vi "Test_WriteValue_NoCaption_Error.vi"(8 "error in (no error)":errorcluster, 11 "TestCase in":refnum<class "TestTerminalCaptionBinding.lvclass">) -> (0 "error out":errorcluster, 3 "TestCase out":refnum<class "TestTerminalCaptionBinding.lvclass">)   [LabVIEW 2017, in "TestTerminalCaptionBinding.lvclass"]
uses:
  TestTerminalCaptionBinding.lvclass
  Source/Concrete/TerminalCaptionBinding/TerminalCaptionBinding.lvclass
  C:/Git/composed-transport/Source/ITransport/ITransport.lvclass
  Source/ITransport/ITransport.lvclass
panel:
  out "Return Error":errorcluster
  in  "Numeric":dbl
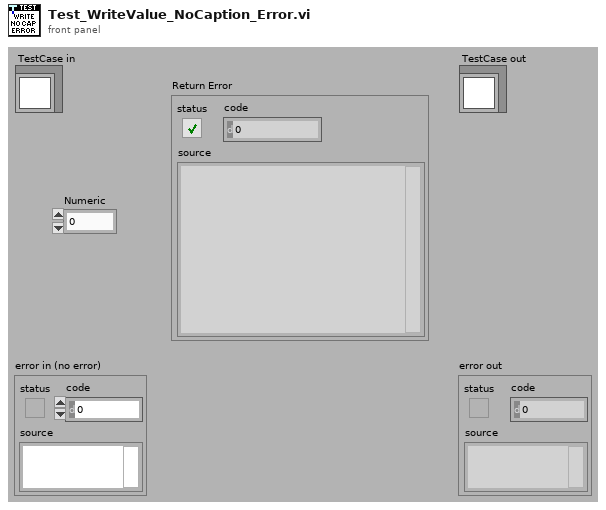
[diagram p1: front panel]
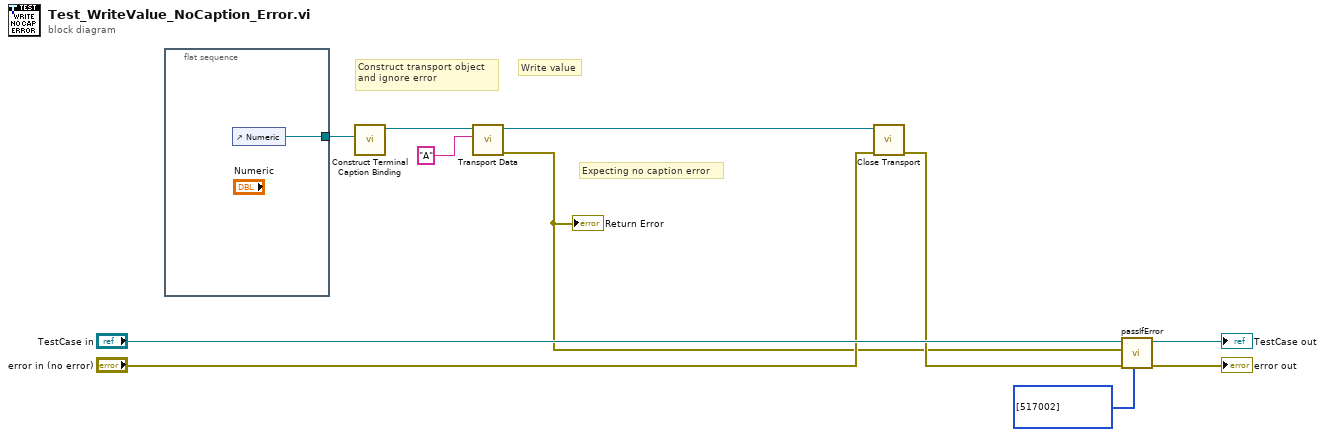
[diagram p0: block diagram]
diagram:
  # "Write value"
  # "Expecting no caption error"
  # "Construct transport object\nand ignore error"
  n1 = flat-sequence {
    tunnel: [w12] -> w7
    frame #0 {
      n2 = control-ref of="Numeric"() -> (w12:refnum<vi>)
    }
  }
  n3 = call "Construct Terminal Caption Binding.vi"("Ctl Refnum"=w7) -> ("TerminalCaptionBinding"=w8:refnum<class "TerminalCaptionBinding.lvclass">)  [unwired: 9 in, 1 out]
  n4 = call "Transport Data.vi"("Value"="A", "ITransport in"=w8) -> ("error out"=w3:errorcluster, "ITransport out"=w4:refnum<class "TerminalCaptionBinding.lvclass">)  [unwired: 8 in]
  "Return Error" <- w3
  n5 = call-dynamic "Close Transport.vi"("error in (no error)"="error in (no error)", "ITransport in"=w4) -> ("error out"=w5:errorcluster)  [unwired: 9 in]
  n6 = call-dynamic "passIfError.vi"("passing error codes (default = any error code)"=i32[] [517002], "error in (no error)"=w5, "error"=w3, "TestCase in"="TestCase in") -> ("error out"=→"error out":errorcluster, "TestCase out"=→"TestCase out":refnum<class "TestTerminalCaptionBinding.lvclass">)  [unwired: 6 in]
